vi "Delete From Array.vi"() -> ()   [LabVIEW 2012]
panel:
  out "Deleted Portion":dbl[][](array[numeric])
  out "Deleted Portion":dbl[](array[numeric])
  out "Output 2D Array":dbl[][](array[numeric])
  out "Output 1D Array":dbl[](array[numeric])
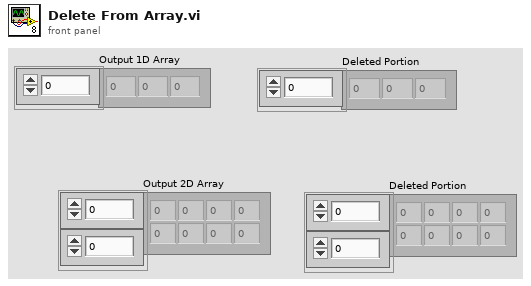
[diagram p1: front panel]
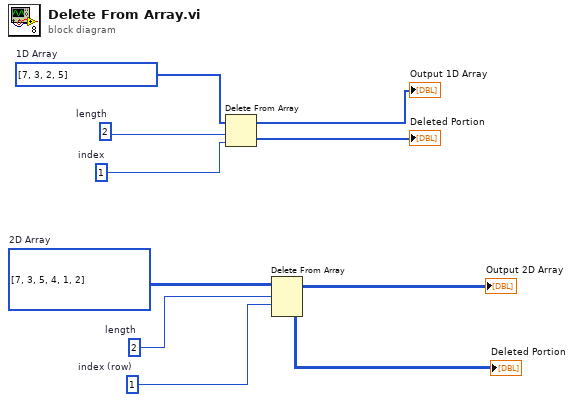
[diagram p0: block diagram]
diagram:
  w2 = 1  # index (row)
  w3 = 2  # length
  w5 = 1  # index
  w6 = 2  # length
  w8 = i32[][] [[7, 3, 5], [4, 1, 2]]  # 2D Array
  w10 = i32[] [7, 3, 2, 5]  # 1D Array
  n1 = Delete From Array "Delete From Array"(array=w10, length=w6, index=w5) -> (deleted portion=→"Deleted Portion":i32[], array with subset deleted=→"Output 1D Array":i32[])
  n2 = Delete From Array "Delete From Array"(array=w8, length=w3, index (row)=w2) -> (deleted portion=→"Deleted Portion":i32[][], array with subset deleted=→"Output 2D Array":i32[][])  [unwired: 1 in]
